vi "Test Process within App Log Info Message.vi"(8 "error in (no error)":errorcluster, 11 "Test Case In":refnum<class "Logger Test.lvclass">) -> (0 "error out":errorcluster, 3 "Test Case Out":refnum<class "Logger Test.lvclass">)   [LabVIEW 2020, in "Logger Test.lvclass"]
uses:
  Logger Test.lvclass
  C:/Program Files (x86)/National Instruments/LabVIEW 2020/vi.lib/Astemes/LUnit/Test Case.lvclass
  source/Framework Test Suite/Mock Log Handler/Mock Log Handler.lvclass
  C:/Git/astemes-triarc-framework/source/Framework/Logging/Logging.lvclass
  source/Framework/Application/Application.lvclass
  C:/Git/astemes-triarc-framework/source/Framework/Process/Process.lvclass
  source/Framework Test Suite/Mock Process/Mock Process.lvclass
  source/Framework/Process/Process.lvclass/Process.ctl
  source/Framework/Application/Application.lvclass/Application.ctl
  <vilib>/Astemes/LUnit/Test Case.lvclass/Test Case.ctl
  <vilib>/Astemes/LUnit/LUnit Assertion Result.lvclass/LUnit Assertion Result.ctl
  <vilib>/Astemes/LUnit/LUnit Test Case Result.lvclass/LUnit Test Case Result.ctl
  <vilib>/Astemes/LUnit/LUnit Method Result.lvclass/LUnit Method Result.ctl
  source/Framework/Process/Public/Lifecycle/Get Lifecycle State.vi
  source/Framework/Process/Protected/Messaging/Enqueue Message.vi
  source/Framework/Application/Private/Add Process to Map.vi
  source/Framework/Application/Private/Start Idle Processes if Running.vi
  source/Framework/Application/Private/Throw Error If Process Already in App.vi
  source/Framework/Process/Protected/SubVIs/Set Context.vi
  source/Framework/Process/Private/SubVIs/Wait for finish.vi
  source/Framework/Process/Private/SubVIs/Set Lifecycle State.vi
  <vilib>/Astemes/LUnit/Palette/Pass If Equal.vi/cbf50e99-f124-4847-863a-8e9794d3dede.vi
  source/Framework/Process/Private/SubVIs/Handle Debug Data.vi
  source/Framework/Application/Public/Get Process.vi
  source/Framework/Process/Public/Lifecycle/Leave Process Loop.vi
  <vilib>/Astemes/LUnit/Palette/Pass.vi
  <vilib>/Astemes/LUnit/Palette/Fail.vi
  <vilib>/Astemes/LUnit/Compare Variants.vi
  <vilib>/Astemes/LUnit/Describe Comparison.vi
  <vilib>/Astemes/LUnit/Set Assertion Type.vi
  source/Framework/Logging/Log Debug.vi
  <vilib>/AdvancedString/1D String Array to Delimited String.vi
  <vilib>/Utility/High Resolution Relative Seconds.vi
  source/Framework/Application/Private/Retrieve Process from App.vi
  source/Framework/Application/Private/Parse Process Name.vi
  source/Framework/Application/Private/Get Process from Map.vi
  <vilib>/Astemes/LUnit/Add test result.vi
  <vilib>/Astemes/LUnit/LUnit Write Passed.vi
  <vilib>/Astemes/LUnit/LUnit Write Message.vi
  <vilib>/Astemes/LUnit/LUnit Write Description.vi
  <vilib>/Astemes/LUnit/Variant to string.vi
  <vilib>/Astemes/LUnit/LUnit Write Assertion Type.vi
  source/Framework/Process/Protected/Messaging/Request Message.vi
  <vilib>/AdvancedString/Delimited String to 1D String Array.vi
  <vilib>/Astemes/LUnit/LUnit Record Assertion Result.vi
  source/Framework/Process/Private/SubVIs/Enqueue Request Message.vi
  <vilib>/Astemes/LUnit/LUnit Aggregate Assertion Results.vi
  <vilib>/Astemes/LUnit/Assertion Result/LUnit Read Status.vi
  <vilib>/Astemes/LUnit/LUnit Read Message.vi
  <vilib>/Astemes/LUnit/LUnit Read Description.vi
  <vilib>/Astemes/LUnit/Method Result/LUnit Merge Status.vi
  <vilib>/Astemes/LUnit/LUnit Concatenate result strings.vi
  <vilib>/Utility/error.llb/Error Cluster From Error Code.vi
  source/Framework/Process/Public/Read Name.vi
  source/Framework/Process/Private/SubVIs/Wait for Response Message.vi
  <vilib>/Utility/Data Type/Get Type Information.vi
  <vilib>/Utility/LVClass/Get LV Class Name.vi
  source/Framework/Process/Process.lvclass
  <vilib>/Astemes/LUnit/LUnit Assertion Result.lvclass
  source/Framework/Logging/Logging.lvclass
  Logger Test.lvclass/Logger Test.ctl
  <vilib>/Astemes/LUnit/Test Case.lvclass
  source/Framework Test Suite/Support/Framework Test Support.lvlib
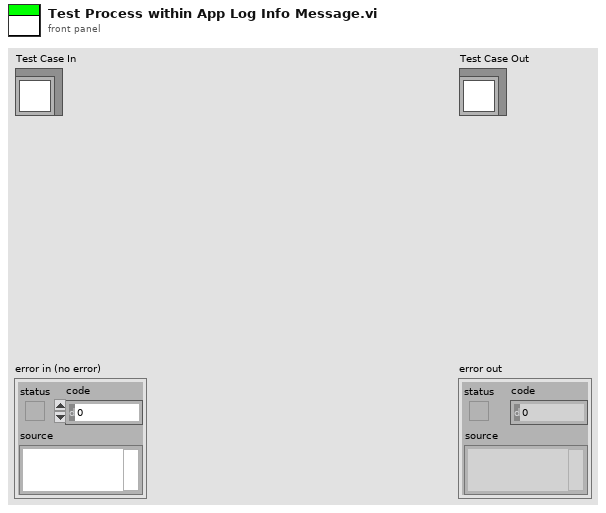
[diagram p1: front panel]
types:
  T1 = typedef "Mock Log Handler.lvclass/Log Entry.ctl" = cluster{"Level":string, "Source":string, "Message":string}
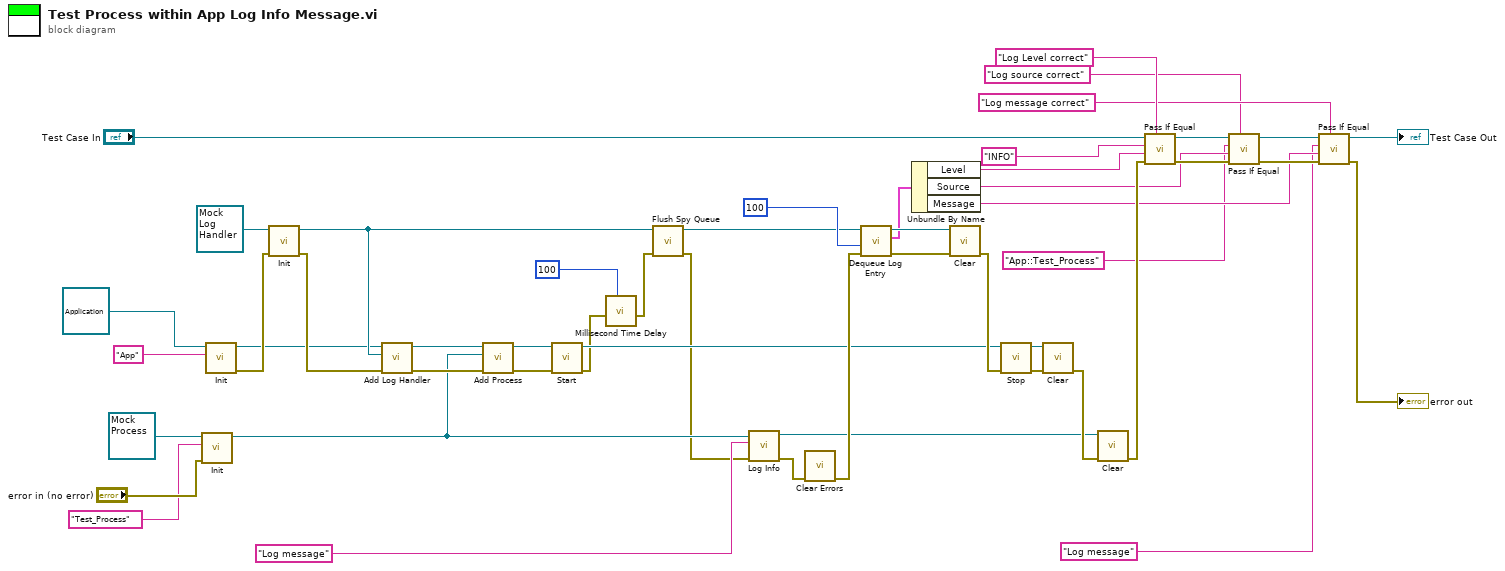
[diagram p0: block diagram]
diagram:
  n1 = call-dynamic "Init.vi"("error in (no error)"="error in (no error)", "Name"="Test_Process", "Mock Process In"=refnum<class "Mock Process.lvclass"> refnum) -> ("Mock Process Out"=w4:refnum<class "Mock Process.lvclass">)  [unwired: 7 in, 1 out]
  n2 = call-dynamic "Init.vi"("Name"="App", "Process In"=refnum<class "Application.lvclass"> refnum ("Application.lvclass")) -> ("error out"=w45:errorcluster, "Process Out"=w2:refnum<class "Application.lvclass">)  [unwired: 8 in]
  n3 = call-dynamic "Init.vi"("error in (no error)"=w45, "Mock Log Handler In"=refnum<class "Mock Log Handler.lvclass"> refnum ("Mock Log Handler.lvclass")) -> ("error out"=w44:errorcluster, "Mock Log Handler Out"=w9:refnum<class "Mock Log Handler.lvclass">)  [unwired: 8 in]
  n4 = call "Add Log Handler.vi"("error in (no error)"=w44, "Log Handler"=w9, "Process In"=w2) -> ("error out"=w19:errorcluster, "Process Out"=w18:refnum<class "Application.lvclass">)  [unwired: 7 in]
  n5 = call "Add Process.vi"("error in (no error)"=w19, "Process"=w4, "Application In"=w18) -> ("error out"=w15:errorcluster, "Application Out"=w1:refnum<class "Application.lvclass">)  [unwired: 7 in]
  n6 = call "Start.vi"("error in (no error)"=w15, "Process In"=w1) -> ("error out"=w7:errorcluster, "Process Out"=w11:refnum<class "Application.lvclass">)  [unwired: 7 in, 1 out]
  n7 = call "Millisecond Time Delay.vi"("milliseconds to wait"=u32 100, "error in (no error)"=w7) -> ("error out"=w6:errorcluster)  [unwired: 7 in]
  n8 = call "Flush Spy Queue.vi"("error in (no error)"=w6, "Mock Log Handler in"=w9) -> ("error out"=w3:errorcluster, "Mock Log Handler out"=w8:refnum<class "Mock Log Handler.lvclass">)  [unwired: 7 in, 1 out]
  n9 = call "Log Info.vi"("error in (no error)"=w3, "Message"="Log message", "Logging In"=w4) -> ("error out"=w25:errorcluster, "Logging Out"=w12:refnum<class "Mock Process.lvclass">)  [unwired: 7 in]
  n10 = call <vilib>:"Clear Errors.vi"("error in (no error)"=w25) -> ("error out"=w24:errorcluster)  [unwired: 5 in, 1 out]
  n11 = call "Dequeue Log Entry.vi"("error in (no error)"=w24, "timeout in ms (-1)"=100, "Mock Log Handler in"=w8) -> ("error out"=w42:errorcluster, "Entry"=w39:T1, "Mock Log Handler out"=w43:refnum<class "Mock Log Handler.lvclass">)  [unwired: 5 in, 1 out]
  n12 = Unbundle By Name(w39) -> ("Level"=w38:string, "Source"=w28:string, "Message"=w27:string)
  n13 = call-dynamic "Clear.vi"("error in (no error)"=w42, "Mock Log Handler In"=w43) -> ("error out"=w40:errorcluster)  [unwired: 9 in]
  n14 = call "Stop.vi"("error in (no error)"=w40, "Process In"=w11) -> ("error out"=w14:errorcluster, "Process Out"=w13:refnum<class "Application.lvclass">)  [unwired: 7 in, 1 out]
  n15 = call-dynamic "Clear.vi"("error in (no error)"=w14, "Application In"=w13) -> ("error out"=w47:errorcluster)  [unwired: 9 in]
  n16 = call-dynamic "Clear.vi"("error in (no error)"=w47, "Mock Process In"=w12) -> ("error out"=w32:errorcluster)  [unwired: 9 in]
  n17 = call <vilib>:"Pass If Equal.vi"("Description"="Log Level correct", "error in (no error)"=w32, "Actual"=w38, "Expected"="INFO", "LUnit Test Case In"="Test Case In") -> ("error out"=w34:errorcluster, "LUnit Test Case Out"=w49:refnum<class "Logger Test.lvclass">)  [unwired: 5 in]
  n18 = call <vilib>:"Pass If Equal.vi"("Description"="Log source correct", "error in (no error)"=w34, "Actual"=w28, "Expected"="App::Test_Process" ("Name"), "LUnit Test Case In"=w49) -> ("error out"=w33:errorcluster, "LUnit Test Case Out"=w36:refnum<class "Logger Test.lvclass">)  [unwired: 5 in]
  n19 = call <vilib>:"Pass If Equal.vi"("Description"="Log message correct", "error in (no error)"=w33, "Actual"=w27, "Expected"="Log message" ("Message"), "LUnit Test Case In"=w36) -> ("error out"=→"error out":errorcluster, "LUnit Test Case Out"=→"Test Case Out":refnum<class "Logger Test.lvclass">)  [unwired: 5 in]
